vi "list_documents.vi"(0 "Device  In":T2, 5 "error in":errorcluster) -> (12 "Comm":T1, 13 "Document list":string[][](array[string]), 14 "Device Out":T2, 19 "error out":errorcluster)   [LabVIEW 2019]
uses:
  <userlib>/IoT Devices/_subVIs/HTTPComm.ctl
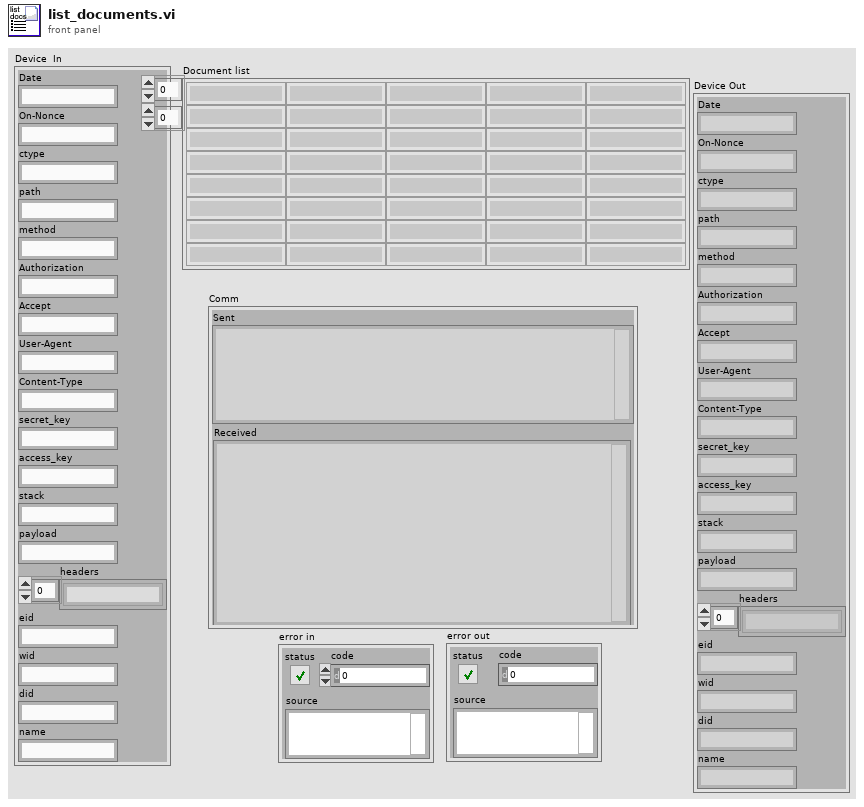
[diagram p1: front panel]
types:
  T1 = typedef "HTTPComm.ctl" = cluster{"url":string, "sent headers":string, "sent body":string, "headers":string, "body":string, "Sent":string, "Received":string}
  T2 = cluster{"Date":string, "On-Nonce":string, "ctype":string, "path":string, "method":string, "Authorization":string, "Accept":string, "User-Agent":string, "Content-Type":string, "secret_key":string, "access_key":string, "stack":string, "payload":string, "headers":string[], "eid":string, "wid":string, "did":string, "name":string}
  T3 = cluster{"items":cluster{"resourceType":string, "id":string, "name":string, "defaultWorkspace":cluster{"id":string}}[]}
  T4 = cluster{"resourceType":string, "id":string, "name":string, "defaultWorkspace":cluster{"id":string}}[]
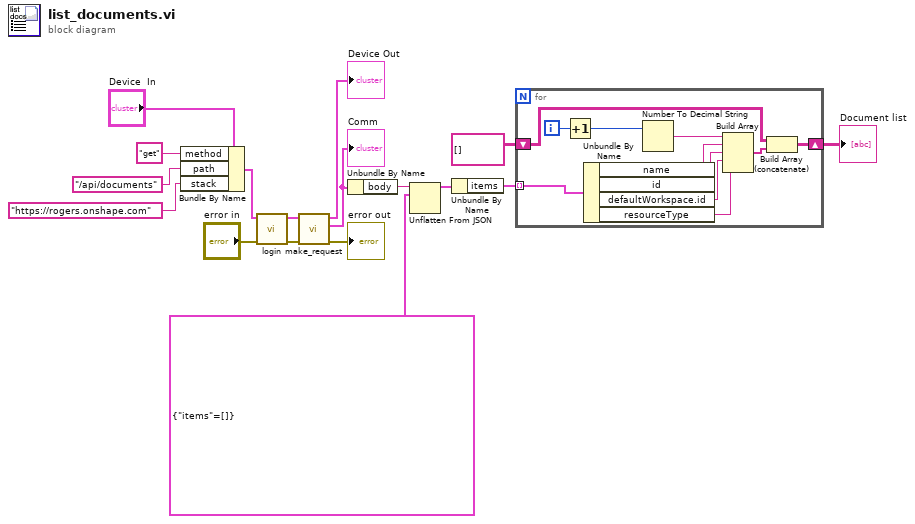
[diagram p0: block diagram]
diagram:
  n1 = Bundle By Name(cluster="Device  In", "method"="get" ("Method"), "path"="/api/documents" ("payload"), "stack"="https://rogers.onshape.com" ("stacks")) -> (w2:T2)
  n2 = call "login.vi"("error in"="error in", "Device In"=w2) -> ("error out"=w3:errorcluster, "Device Out"=w1:T2)  [unwired: 8 in]
  n3 = call "make_request.vi"("Error in"=w3, "Device In"=w1) -> ("error out"=→"error out":errorcluster, "Comm"=w11:T1, "Device Out"=→"Device Out":T2)  [unwired: 7 in]
  "Comm" <- w11
  n4 = Unbundle By Name(w11) -> ("body"=w10:string)
  n5 = Unflatten From JSON(JSON string=w10, type and defaults=T3 {"items"=[]}) -> (value=w8:T3)  [unwired: 5 in, 1 out]
  n6 = Unbundle By Name(w8) -> ("items"=w7:T4)
  n7 = for {
    tunnel: w7 -> [w28] mode=indexing
    shift-right: [w26] -> w5
    shift-left: string[][] [] -> [w27]
    i -> [w21]
    n8 = Increment(x=w21) -> (x+1=w20:i32)
    n9 = Unbundle By Name(w28) -> ("name"=w25:string, "id"=w24:string, "defaultWorkspace.id"=w23:string, "resourceType"=w18:string)
    n10 = Number To Decimal String(number=w20) -> (decimal integer string=w19:string)  [unwired: 1 in]
    n11 = Build Array(w19, w25, w24, w23, w18) -> (w22:string[])
    n12 = Build Array (concatenate)(w27, w22) -> (w26:string[][])
  }
  "Document list" <- w5
